vi "music-learner-mcu.vi"() -> ()   [LabVIEW 2015]
panel:
  in  "Weights L2N1":dbl[](array[numeric])
  out "Neural Net Output":dbl
  in  "Toggle Mode":bool
  out "error out":errorcluster
  in  "Stop":bool
  out "Inference Mode":bool
  out "Learning Mode":bool
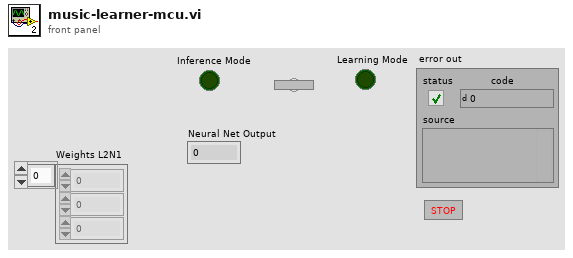
[diagram p1: front panel]
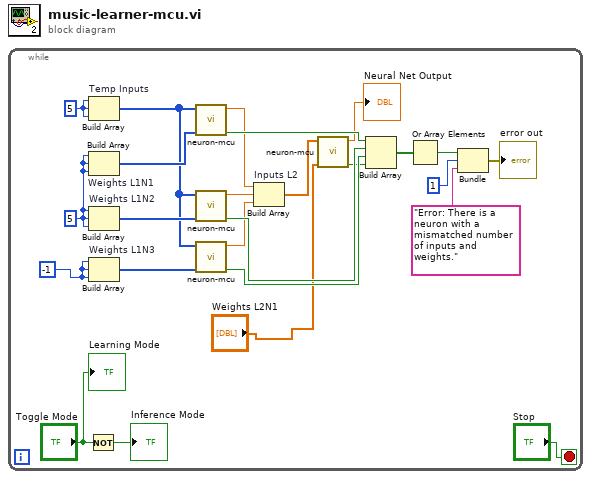
[diagram p0: block diagram]
diagram:
  n1 = while {
    stop <- "Stop" stop-if-true
    w1 = -1
    w15 = 5
    w18 = 5
    n2 = Not(x="Toggle Mode") -> (.not. x?=→"Inference Mode":bool)
    n3 = Build Array "Temp Inputs"(w18, w18, w18) -> (w14:i32[])
    n4 = Build Array "Weights L1N1"(w15, w15, w15) -> (w19:i32[])
    n5 = Build Array "Weights L1N2"(w15, w15, w15) -> (w17:i32[])
    n6 = Build Array "Weights L1N3"(w1, w1, w1) -> (w16:i32[])
    n7 = call "neuron-mcu.vi"("Weights"=w19, "Inputs"=w14) -> ("Error?"=w13:bool, "Output"=w8:dbl)  [unwired: 8 in]
    n8 = call "neuron-mcu.vi"("Weights"=w17, "Inputs"=w14) -> ("Error?"=w12:bool, "Output"=w7:dbl)  [unwired: 8 in]
    n9 = call "neuron-mcu.vi"("Weights"=w16, "Inputs"=w14) -> ("Error?"=w11:bool, "Output"=w6:dbl)  [unwired: 8 in]
    n10 = Build Array "Inputs L2"(w8, w7, w6) -> (w5:dbl[])
    n11 = call "neuron-mcu.vi"("Weights"="Weights L2N1", "Inputs"=w5) -> ("Error?"=w4:bool, "Output"=→"Neural Net Output":dbl)  [unwired: 8 in]
    n12 = Build Array(w13, w12, w11, w4) -> (w10:bool[])
    n13 = Or Array Elements(Boolean array=w10) -> (logical OR=w9:bool)
    n14 = Bundle(w9, 1, "Error: There is a neuron with a mismatched number of inputs and weights.") -> (→"error out":errorcluster)  [unwired: 1 in]
    "Learning Mode" <- "Toggle Mode"
  }
